vi "Open file with default application complicated.vi"(0 "file path":path, 11 "error in":errorcluster) -> (4 "command line":string, 15 "error out":errorcluster)   [LabVIEW 2013]
uses:
  <vilib>/Utility/error.llb/whitespace.ctl
  resource/Public/Subs/ViServer/Message Logger Fuction.ctl
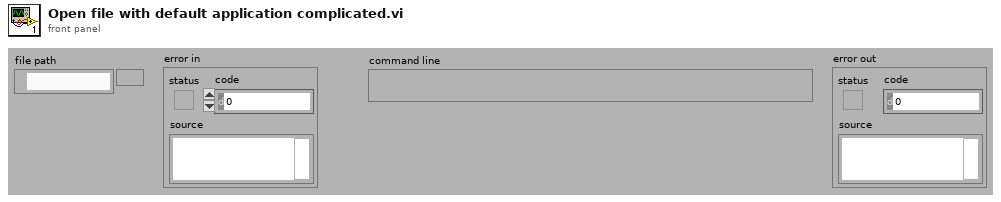
[diagram p1: front panel]
types:
  T1 = typedef "Message Logger Fuction.ctl" = enum16{"set config", "log messages", "log errors", "log & del err"}
  T2 = typedef "whitespace.ctl" = u16
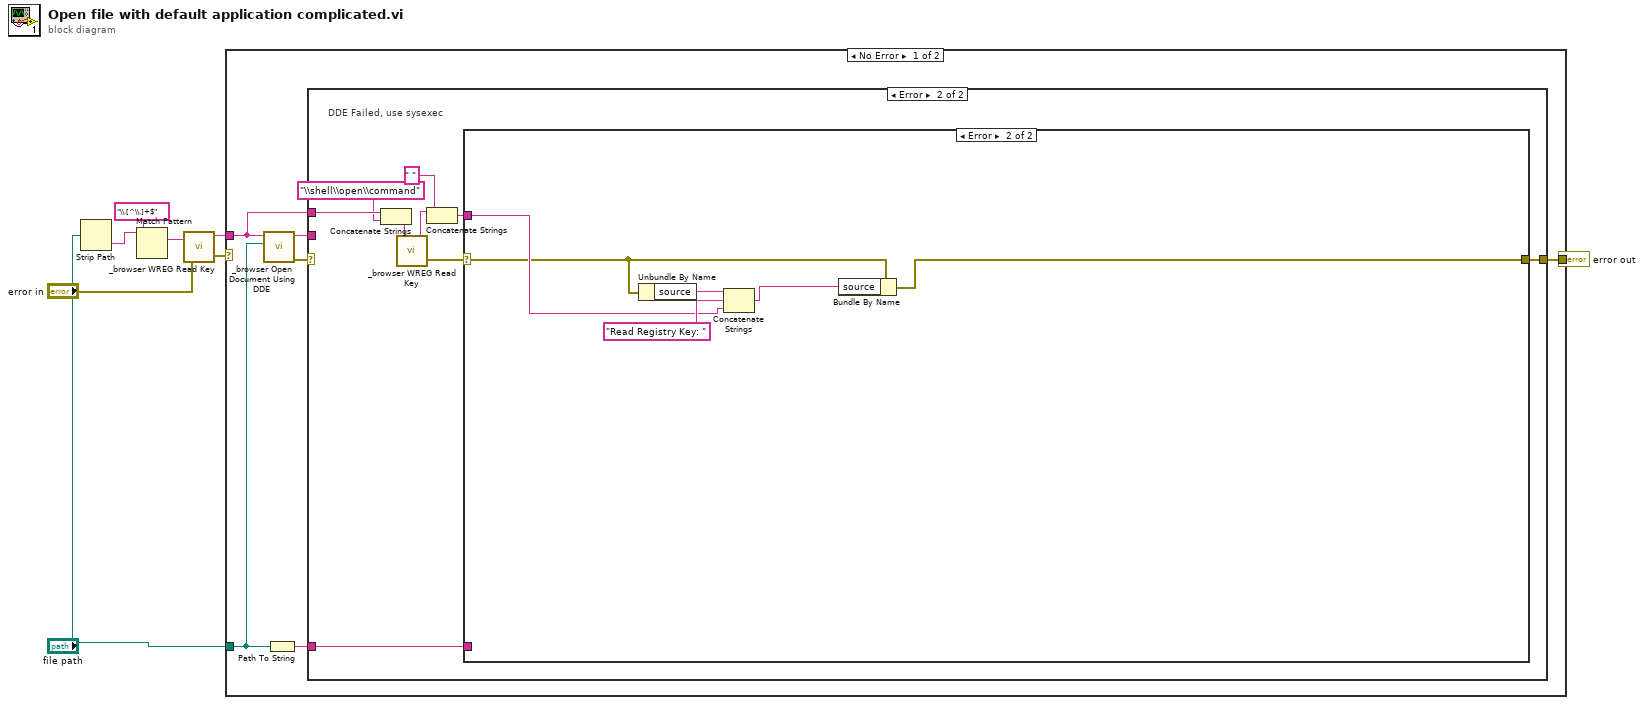
[diagram p0: block diagram]
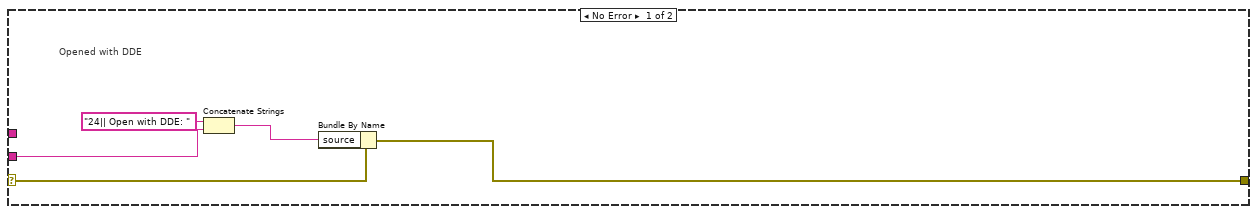
[diagram p2: hidden frame]
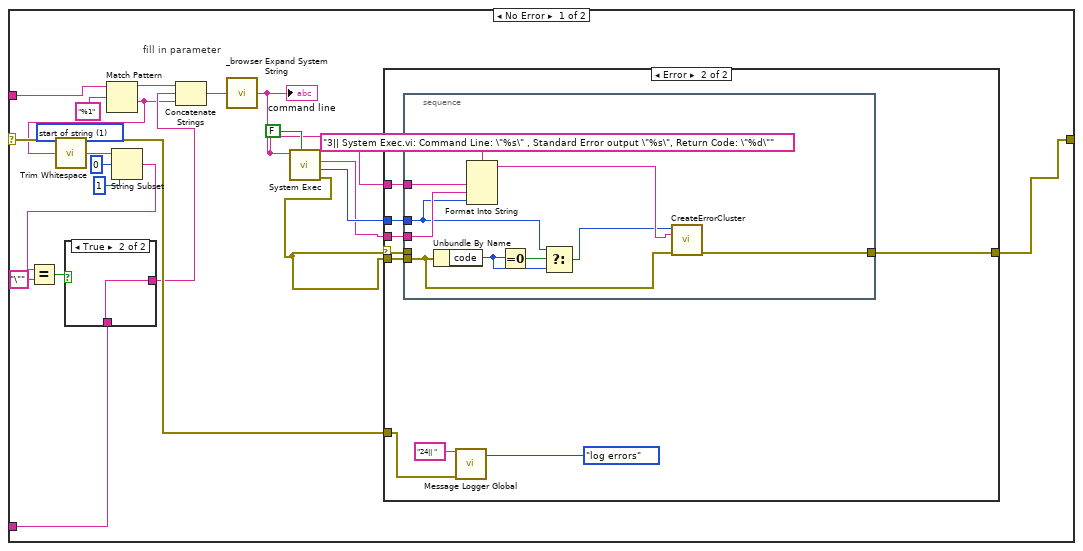
[diagram p3: hidden frame]
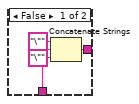
[diagram p4: hidden frame]
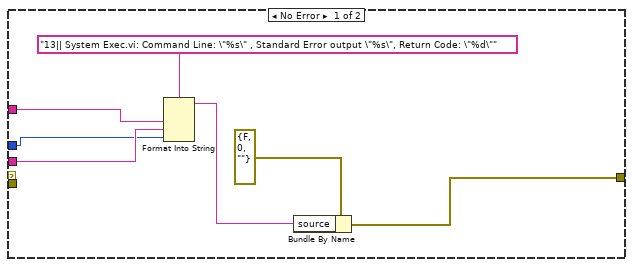
[diagram p5: hidden frame]
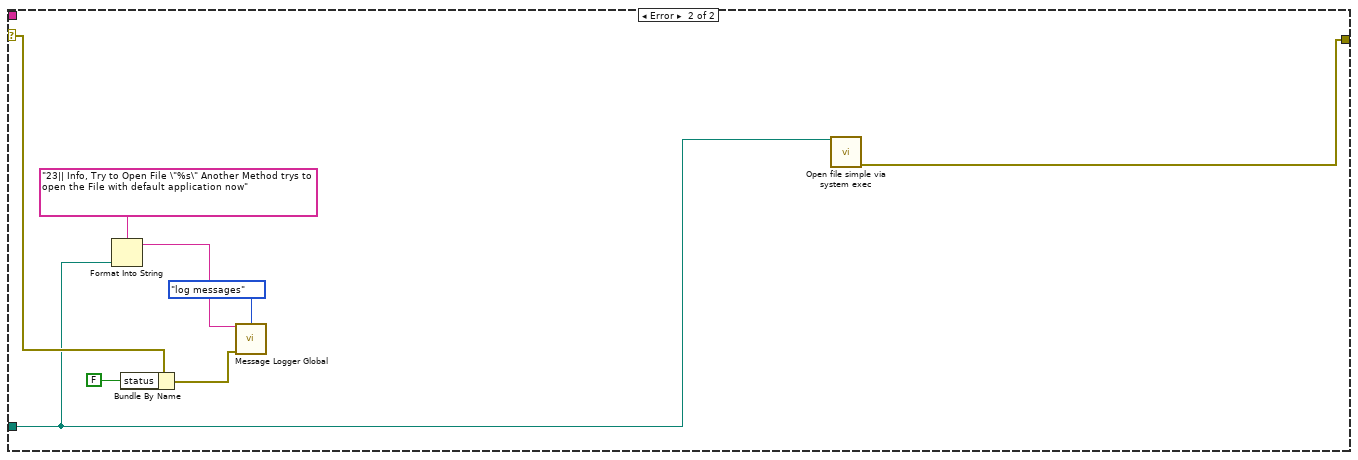
[diagram p6: hidden frame]
diagram:
  n1 = Strip Path(path="file path") -> (name=w1:string)  [unwired: 1 out]
  n2 = Match Pattern(string=w1, regular expression="\\.[^\\.]+$") -> (match substring=w3:string)  [unwired: 1 in, 3 out]
  n3 = call <vilib>:"_browser WREG Read Key.vi"("error in (no error)"="error in", "subkey"=w3) -> ("error out"=w8:errorcluster, "string data"=w6:string)
  n4 = case shown="No Error" w8 {
    selector: w8 -> [_ w92]
    tunnel: [w14 w94] -> w5
    tunnel: w6 -> [w13 _]
    tunnel: "file path" -> [w9 w88]
    frame No Error {
      n5 = call "_browser Open Document Using DDE.vi"("document"=w9, "service"=w13) -> ("error out"=w11:errorcluster, "DDE String"=w10:string)  [unwired: 4 in]
      n6 = Path To String(path=w9) -> (string=w12:string)
      n7 = case shown="Error" w11 {
        selector: w11 -> [w19 _]
        tunnel: [w18 w28] -> w14
        tunnel: w13 -> [_ w27]
        tunnel: w12 -> [_ w24]
        tunnel: w10 -> [w15 _]
        frame No Error {
          # "Opened with DDE"
          n8 = Concatenate Strings("24|| Open with DDE: " ("string"), w15) -> (w17:string)
          n9 = Bundle By Name(cluster=w19, "source"=w17) -> (w18:errorcluster)
        }
        frame Error {
          # "DDE Failed, use sysexec"
          n10 = Concatenate Strings(w27, "\\shell\\open\\command" ("subkey")) -> (w25:string)
          n11 = call <vilib>:"_browser WREG Read Key.vi"("subkey"=w25) -> ("error out"=w23:errorcluster, "string data"=w21:string)  [unwired: 1 in]
          n12 = Concatenate Strings(w21, " " ("string")) -> (w22:string)
          n13 = case shown="Error" w23 {
            selector: w23 -> [w44 w83]
            tunnel: w24 -> [w45 _]
            tunnel: [w40 w82] -> w28
            tunnel: w22 -> [w33 w84]
            frame No Error {
              w31 = T2 1 items=["both", "start of string", "end of string"] ("location (both)")
              # "fill in parameter"
              n14 = Match Pattern(string=w33, regular expression="%1") -> (before substring=w48:string, after substring=w30:string)  [unwired: 1 in, 2 out]
              n15 = call <vilib>:"Trim Whitespace.vi"("string"=w30, "location (both)"=w31) -> ("trimmed string"=w32:string)
              n16 = String Subset(string=w32, offset (0)=0, length (rest)=1 ("length (rest)")) -> (substring=w37:string)
              n17 = Equal?(x=w37, y="\"") -> (x = y?=w38:bool)
              n18 = case shown="True" w38 {
                tunnel: w45 -> [w53 w54]
                tunnel: [w50 w54] -> w39
                frame False {
                  n19 = Concatenate Strings("\"" ("string"), w53, "\"" ("string")) -> (w50:string)
                }
                frame True {
                }
              }
              n20 = Concatenate Strings(w48, w39, w30) -> (w47:string)
              n21 = call <vilib>:"_browser Expand System String.vi"("system string"=w47) -> ("expanded string"=w43:string)
              "command line" <- w43
              n22 = call <vilib>:"System Exec.vi"("wait until completion? (T)"=FALSE, "command line"=w43) -> ("error out"=w29:errorcluster, "return code"=w42:i32, "standard error"=w41:string)  [unwired: 6 in, 1 out]
              n23 = case shown="Error" w29 {
                selector: w29 -> [_ w70]
                tunnel: [w60 w69] -> w40
                tunnel: w41 -> [w58 w68]
                tunnel: w43 -> [w59 w67]
                tunnel: w42 -> [w55 w66]
                tunnel: w29 -> [_ w65]
                tunnel: w44 -> [_ w62]
                frame No Error {
                  n24 = Format Into String(format string="13|| System Exec.vi: Command Line: \"%s\" , Standard Error output \"%s\", Return Code: \"%d\"", w59, w58, w55) -> (resulting string=w57:string)  [unwired: 2 in, 1 out]
                  n25 = Bundle By Name(cluster=errorcluster {"status"=FALSE, "code"=0, "source"=""} ("error out 2"), "source"=w57) -> (w60:errorcluster)
                }
                frame Error {
                  n26 = stacked-sequence {
                    tunnel: w70 -> [_]
                    tunnel: [w80] -> w69
                    tunnel: w68 -> [w79]
                    tunnel: w67 -> [w77]
                    tunnel: w66 -> [w71]
                    tunnel: w65 -> [w72]
                    frame #0 {
                      n27 = Unbundle By Name(w72) -> ("code"=w74:i32)
                      n28 = Format Into String(format string="3|| System Exec.vi: Command Line: \"%s\" , Standard Error output \"%s\", Return Code: \"%d\"", w77, w79, w71) -> (resulting string=w76:string)  [unwired: 2 in, 1 out]
                      n29 = Equal To 0?(x=w74) -> (x = 0?=w75:bool)
                      n30 = Select(t=w71, s=w75, f=w74) -> (s? t:f=w73:i32)
                      n31 = call "CreateErrorCluster.vi"("Error Code"=w73, "Additional description"=w76, "error in"=w72) -> ("error out"=w80:errorcluster)  [unwired: 12 in]
                    }
                  }
                  n32 = call "Message Logger Global.vi"("Message in"="24|| ", "Message Logger Function"=Message_Logger_Fuction."log errors", "error in (no error)"=w62) -> ()  [unwired: 12 in, 1 out]
                }
              }
            }
            frame Error {
              n33 = Unbundle By Name(w83) -> ("source"=w86:string)
              n34 = Concatenate Strings(w86, "Read Registry Key: " ("string"), w84) -> (w81:string)
              n35 = Bundle By Name(cluster=w83, "source"=w81) -> (w82:errorcluster)
            }
          }
        }
      }
    }
    frame Error {
      n36 = Format Into String(format string="23|| Info, Try to Open File \"%s\" Another Method trys to open the File with default application now" ("Message in"), w88) -> (resulting string=w87:string)  [unwired: 2 in, 1 out]
      n37 = Bundle By Name(cluster=w92, "status"=FALSE) -> (w91:errorcluster)
      n38 = call "Message Logger Global.vi"("Message in"=w87, "Message Logger Function"=Message_Logger_Fuction."log messages", "error in (no error)"=w91) -> ()  [unwired: 12 in, 1 out]
      n39 = call "Open file simple via system exec.vi"("file path"=w88) -> ("error out"=w94:errorcluster)  [unwired: 13 in, 1 out]
    }
  }
  "error out" <- w5
